vi "JoyToFps.vi"(11 "JoystickInput":dbl) -> (3 "Fps":dbl)   [LabVIEW 2020]
doc: "Converts JoystickInput to Fps on top and Fps to joystick on bottom"
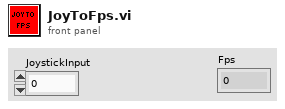
[diagram p1: front panel]
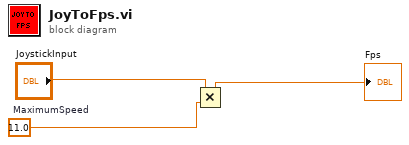
[diagram p0: block diagram]
diagram:
  w2 = 11.0  # MaximumSpeed
  n1 = Multiply(x="JoystickInput", y=w2) -> (x*y=→"Fps":dbl)
